vi "Write Color.vi"(5 "Color":u32(colorbox), 9 "Cluster in":refnum<class "Cluster.lvclass">) -> (3 "Cluster out":refnum<class "Cluster.lvclass">)   [LabVIEW 2014, in "Cluster.lvclass"]
uses:
  Cluster.lvclass
  Cluster.lvclass/Cluster.ctl
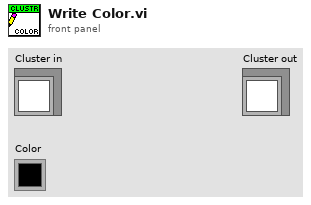
[diagram p1: front panel]
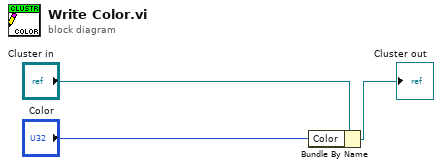
[diagram p0: block diagram]
diagram:
  n1 = Bundle By Name(cluster="Cluster in", "Color"="Color") -> (→"Cluster out":refnum<class "Cluster.lvclass">)
